vi "Populate Available Wfms.vi"(8 "error in":errorcluster, 9 "ListBox Variant":variant, 10 "CD Settings":T1={"CD Task Dependency"=18446744073709551615, "CD Task Dependency Ref"=18446744073709551615, "CD Task Available Wfms"=[], "CD Task Selected Wfms"=[], "Buffer Length (s)"=0.0, "Buffer Length (samples)"=0, "Single-point Enabled"=FALSE, "Running Average Enabled"=FALSE, "Task Rate"=0.0} {"CD Task Dependency Ref" format="%.0x"; "CD Task Dependency" format="%.0x"}, 11 "CustomDevice Ref":T2 format="%.0x") -> (0 "error out":errorcluster, 1 "ListBox Variant":variant, 2 "CD Settings out":T1={"CD Task Dependency"=18446744073709551615, "CD Task Dependency Ref"=18446744073709551615, "CD Task Available Wfms"=[], "CD Task Selected Wfms"=[], "Buffer Length (s)"=0.0, "Buffer Length (samples)"=0, "Single-point Enabled"=FALSE, "Running Average Enabled"=FALSE, "Task Rate"=0.0} {"CD Task Dependency Ref" format="%.0x"; "CD Task Dependency" format="%.0x"}, 3 "CustomDevice Ref":T2 format="%.0x")   [LabVIEW 2015, in "Waveform-Processing-Custom-Device System Explorer.lvlib"]
uses:
  Waveform-Processing-Custom-Device System Explorer.lvlib
  <vilib>/NI Veristand/Custom Device API/Custom Device Item Ref.ctl
  Shared/Custom Device Settings.ctl
  NationalInstruments.VeriStand.SystemStorage
  NationalInstruments.VeriStand
  <vilib>/NI Veristand/Custom Device Tools/Custom Device Utility Library/Custom Device Utility Library.lvlib
  <vilib>/NI VeriStand/Custom Device API/Custom Device API.lvlib
  Shared/Waveform-Processing-Custom-Device Shared.lvlib
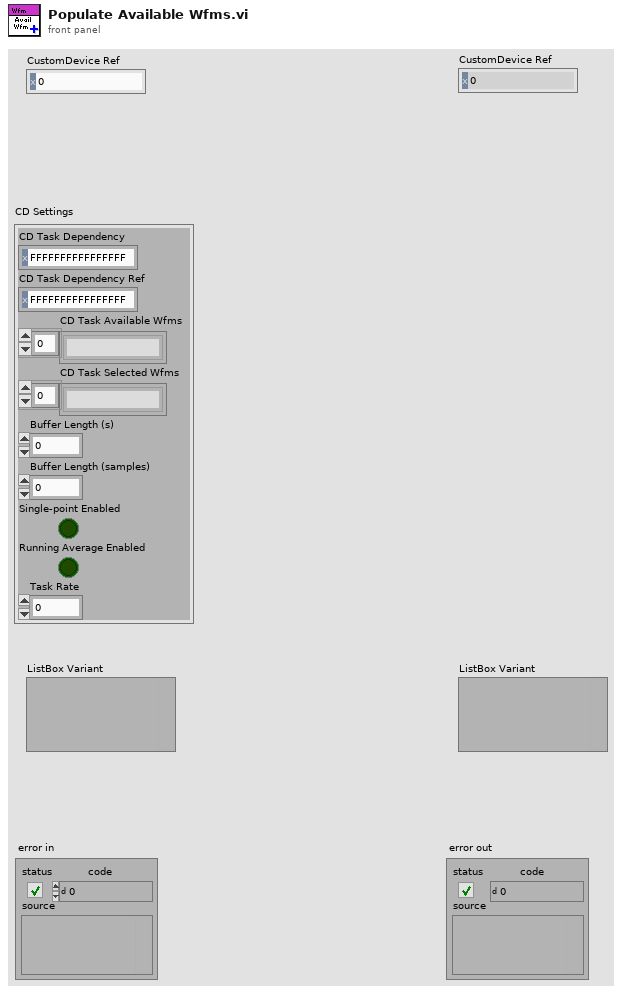
[diagram p1: front panel]
types:
  T1 = typedef "Waveform-Processing-Custom-Device Shared.lvlib/Custom Device Settings.ctl" = cluster{"CD Task Dependency":T2, "CD Task Dependency Ref":T2, "CD Task Available Wfms":string[], "CD Task Selected Wfms":string[], "Buffer Length (s)":dbl, "Buffer Length (samples)":u32, "Single-point Enabled":bool, "Running Average Enabled":bool, "Task Rate":dbl}
  T2 = typedef "Custom Device API.lvlib/Custom Device Item Ref.ctl" = u64
  T3 = typedef "Custom Device API.lvlib/Custom Device Pointer.ctl" = refnum<k24>
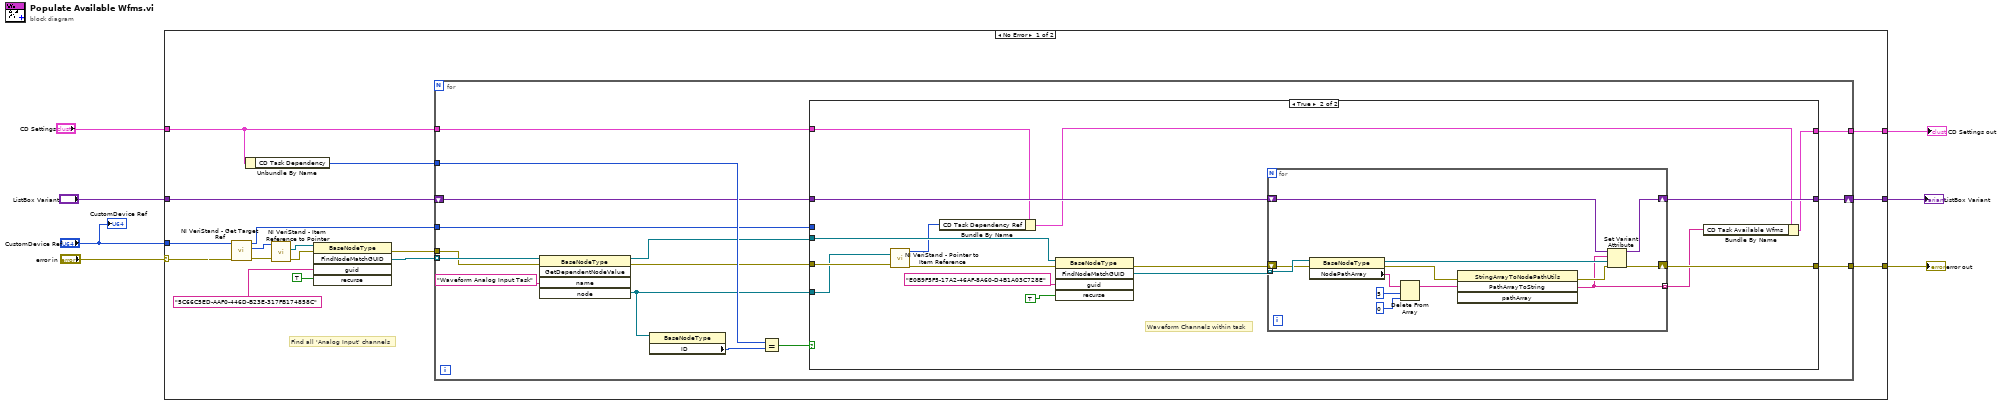
[diagram p0: block diagram]
diagram:
  n1 = case shown="No Error" "error in" {
    selector: "error in" -> [w24 w74]
    tunnel: [w15 w74] -> w4
    tunnel: "CustomDevice Ref" -> [w12 _]
    tunnel: [w14 w73] -> w5
    tunnel: "ListBox Variant" -> [w13 w73]
    tunnel: "CD Settings" -> [w9 w72]
    tunnel: [w8 w72] -> w1
    frame No Error {
      # "Find all 'Analog Input' channels"
      n2 = call <vilib>:"NI VeriStand - Get Target Ref.vi"("error in"=w24, "Item Ref in"=w12) -> ("error out"=w23:errorcluster, "Target Ref"=w22:T2, "Item Ref out"=w11:T2)  [unwired: 6 in, 1 out]
      n3 = Unbundle By Name(w9) -> ("CD Task Dependency"=w10:T2)
      n4 = call <vilib>:"NI VeriStand - Item Reference to Pointer.vi"("error in (no error)"=w23, "Item Ref in"=w22) -> ("error out"=w20:errorcluster, "Node Pointer"=w21:T3)  [unwired: 6 in, 2 out]
      n5 = invoke class="BaseNodeType" method="FindNodeMatchGUID"(reference=w21, error in=w20, "guid"="5C66C5ED-AAF0-446D-B23E-317FB174858C" ("Item GUID"), "recurse"=TRUE ("Find All? (T)")) -> (error out=w16:errorcluster, "FindNodeMatchGUID"=w17:refnum<k24>[])  [unwired: 1 in, 3 out]
      n6 = for {
        tunnel: w10 -> [w39]
        tunnel: w17 -> [w38] mode=indexing
        tunnel: w16 -> [w37]
        tunnel: [w32] -> w15
        shift-right: [w31] -> w14
        shift-left: w13 -> [w30]
        tunnel: w11 -> [w29]
        tunnel: w9 -> [w26]
        tunnel: [w25] -> w8
        n7 = invoke class="BaseNodeType" method="GetDependentNodeValue"(reference=w38, error in=w37, "name"="Waveform Analog Input Task" ("Property Name")) -> (reference out=w27:refnum<k24>, error out=w34:errorcluster, "node"=w28:refnum<k24>)  [unwired: 2 in, 2 out]
        n8 = property class="BaseNodeType"(reference=w28) -> ("ID"=w35:u64)  [unwired: 1 in, 2 out]
        n9 = Equal?(x=w39, y=w35) -> (x = y?=w33:bool)
        n10 = case shown="True" w33 {
          tunnel: w28 -> [_ w50]
          tunnel: w34 -> [w42 w51]
          tunnel: [w42 w54] -> w32
          tunnel: [w41 w53] -> w31
          tunnel: w30 -> [w41 w52]
          tunnel: w29 -> [_ _]
          tunnel: w27 -> [_ w49]
          tunnel: w26 -> [w40 w48]
          tunnel: [w40 w43] -> w25
          frame False {
          }
          frame True {
            # "Waveform Channels within task"
            n11 = call <vilib>:"NI VeriStand - Pointer to Item Reference.vi"("error in (no error)"=w51, "Node Pointer"=w50) -> ("error out"=w46:errorcluster, "Item Ref out"=w47:T2)  [unwired: 8 in]
            n12 = Bundle By Name(cluster=w48, "CD Task Dependency Ref"=w47) -> (w45:T1)
            n13 = invoke class="BaseNodeType" method="FindNodeMatchGUID"(reference=w49, error in=w46, "guid"="E0B9F5F5-17A2-46AF-8A60-D4B1A03C728E", "recurse"=TRUE ("Find All? (T)")) -> (error out=w55:errorcluster, "FindNodeMatchGUID"=w56:refnum<k24>[])  [unwired: 1 in, 3 out]
            n14 = for {
              tunnel: w56 -> [w67] mode=indexing
              shift-right: [w63] -> w53
              shift-left: w52 -> [w62]
              shift-right: [w64] -> w54
              shift-left: w55 -> [w66]
              tunnel: [w59] -> w44 mode=indexing
              n15 = property class="BaseNodeType"(reference=w67, error in=w66) -> (reference out=w61:refnum<k24>, error out=w65:errorcluster, "NodePathArray"=w68:string[])
              n16 = Delete From Array(array=w68, length=5, index=0) -> (array with subset deleted=w71:string[])  [unwired: 1 out]
              n17 = invoke class="StringArrayToNodePathUtils" method="PathArrayToString"(error in=w65, "pathArray"=w71) -> (error out=w60:errorcluster, "PathArrayToString"=w59:string)  [unwired: 2 in, 2 out]
              n18 = Set Variant Attribute(Variant=w62, name=w59, value=w61, error in=w60) -> (Variant out=w63:variant, error out=w64:errorcluster)  [unwired: 1 out]
            }
            n19 = Bundle By Name(cluster=w45, "CD Task Available Wfms"=w44) -> (w43:T1)
          }
        }
      }
    }
    frame Error {
    }
  }
  "error out" <- w4
  "ListBox Variant" <- w5
  "CD Settings out" <- w1
  "CustomDevice Ref" <- "CustomDevice Ref"
